vi "Read (yzb).vi"(7 "Timeout (10000 ms)":u32=10000, 8 "error in (no error)":errorcluster, 11 "VISA resource name":refnum<visa-resource-name>="GPIB0::8::INSTR") -> (0 "error out":errorcluster, 2 "Parameter Values":T1, 3 "VISA resource name out":refnum<visa-resource-name>)   [LabVIEW 2017]
doc: "Reads all the available parameters from the instrument.\n\n<B>Note:</B>\n\nThis VI only reads multiple parameters, not multiple points of the same parameter."
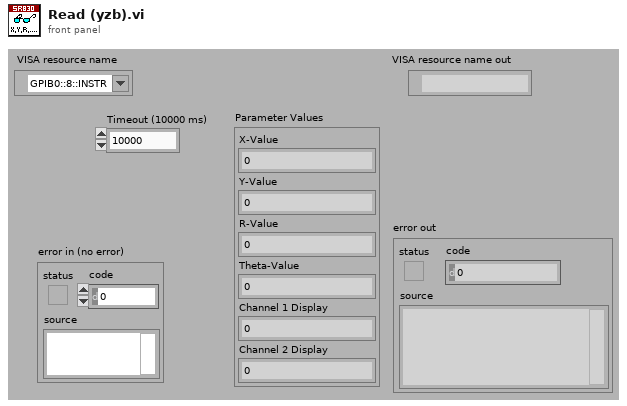
[diagram p1: front panel]
types:
  T1 = cluster{"X-Value":dbl, "Y-Value":dbl, "R-Value":dbl, "Theta-Value":dbl, "Channel 1 Display":dbl, "Channel 2 Display":dbl}
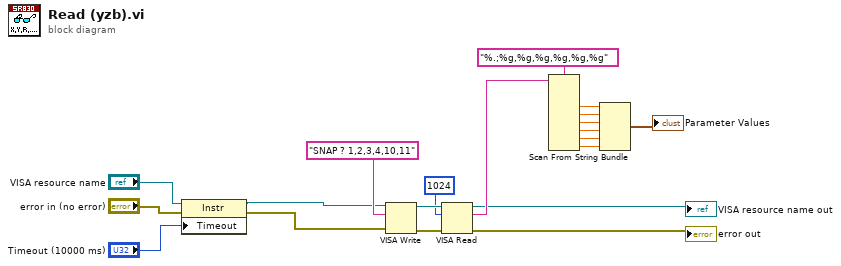
[diagram p0: block diagram]
diagram:
  n1 = property class="Instr"(reference="VISA resource name", error in="error in (no error)", "Timeout"="Timeout (10000 ms)") -> (reference out=w2:refnum<visa-resource-name>, error out=w1:errorcluster)
  n2 = VISA Write(VISA resource name=w2, write buffer="SNAP ? 1,2,3,4,10,11", error in (no error)=w1) -> (VISA resource name out=w19:refnum<visa-resource-name>, error out=w20:errorcluster)  [unwired: 1 out]
  n3 = VISA Read(VISA resource name=w19, byte count=u32 1024, error in (no error)=w20) -> (VISA resource name out=→"VISA resource name out":refnum<visa-resource-name>, read buffer=w5:string, error out=→"error out":errorcluster)  [unwired: 1 out]
  n4 = Scan From String(format string="%.;%g,%g,%g,%g,%g,%g", input string=w5) -> (output 1=w14:dbl, output 2=w13:dbl, output 3=w12:dbl, output 4=w11:dbl, output 5=w7:dbl, output 6=w6:dbl)  [unwired: 8 in, 3 out]
  n5 = Bundle(w14, w13, w12, w11, w7, w6) -> (→"Parameter Values":cluster{dbl, dbl, dbl, dbl, dbl, dbl})  [unwired: 1 in]
